vi "get_data_path.vi"(10 "Dataset directory":path=path "C:/Users/Naomi Tan/Documents/Gillette/ML/STIR_ML_dev/LabView/original_images/IMG_6155.JPG", 11 "Image path":path) -> (2 "Exists":bool, 3 "Dataset path":path)   [LabVIEW 2024]
panel:
  out "Exists 2":bool
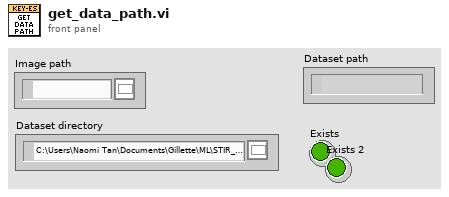
[diagram p1: front panel]
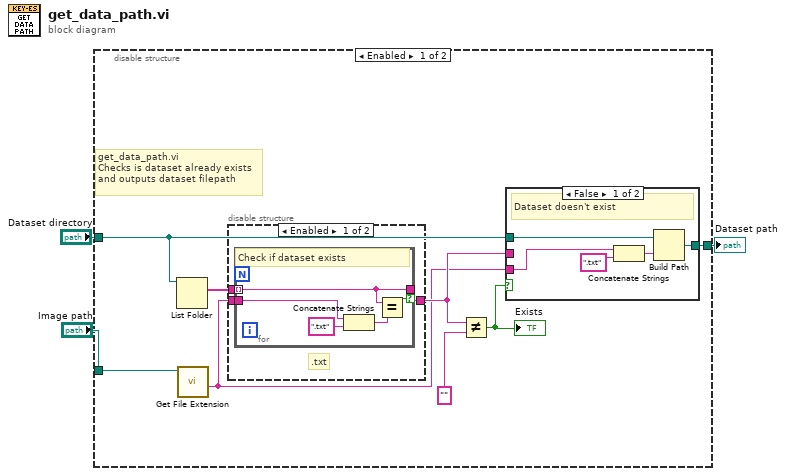
[diagram p0: block diagram]
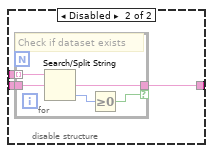
[diagram p2: hidden frame]
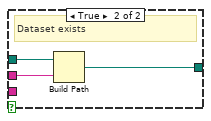
[diagram p3: hidden frame]
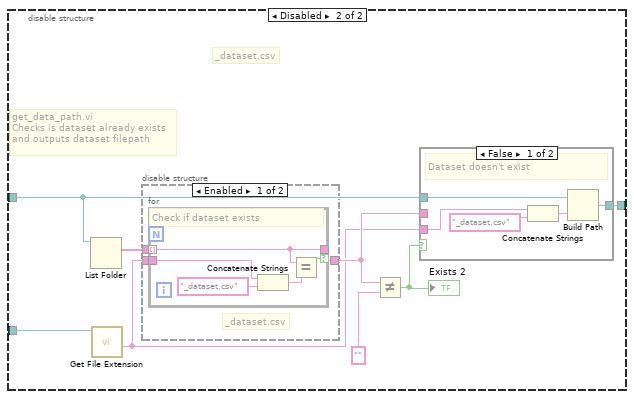
[diagram p4: hidden frame]
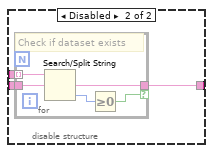
[diagram p5: hidden frame]
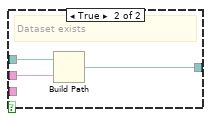
[diagram p6: hidden frame]
diagram:
  n1 = disable-structure shown="Enabled" {
    disable-tunnel: "Image path" -> [w11 w43]
    disable-tunnel: "Dataset directory" -> [w7 w39]
    disable-tunnel: [w4 w36] -> w1
    frame Enabled {
      # "get_data_path.vi\nChecks is dataset already exists\nand outputs dataset filepath"
      n2 = List Folder(path=w7) -> (filenames=w10:string[])  [unwired: 3 in, 3 out]
      n3 = call <vilib>:"Get File Extension.vi"("file"=w11) -> ("filename without extension"=w5:string)  [unwired: 6 in, 4 out]
      n4 = disable-structure shown="Enabled" {
        disable-tunnel: w10 -> [w14 w22]
        disable-tunnel: [w12 w21] -> w6
        disable-tunnel: w5 -> [w13 w20]
        frame Enabled {
          # ".txt"
          n5 = for {
            tunnel: w14 -> [w16] mode=indexing
            tunnel: w13 -> [w18]
            tunnel: [w16] -> w12 if=w15
            # "Check if dataset exists"
            n6 = Concatenate Strings(w18, ".txt" ("string")) -> (w17:string)
            n7 = Equal?(x=w16, y=w17) -> (x = y?=w15:bool)
          }
        }
        frame Disabled {
          n8 = for {
            tunnel: w22 -> [w26] mode=indexing
            tunnel: w20 -> [w27]
            tunnel: [w25] -> w21 if=w23
            # "Check if dataset exists"
            n9 = Search/Split String(string=w26, search string/char (-)=w27) -> (match + rest of string=w25:string, offset of match=w24:i32)  [unwired: 1 in, 1 out]
            n10 = Greater Or Equal To 0?(x=w24) -> (x >= 0?=w23:bool)
          }
        }
      }
      n11 = Not Equal?(x=w6, y="" ("delimiter (\\t)")) -> (x != y?=w8:bool)
      "Exists" <- w8
      n12 = case shown="False" w8 {
        tunnel: w7 -> [w32 w35]
        tunnel: w6 -> [_ w34]
        tunnel: w5 -> [w30 _]
        tunnel: [w28 w33] -> w4
        frame False {
          # "Dataset doesn't exist"
          n13 = Concatenate Strings(w30, ".txt" ("string")) -> (w31:string)
          n14 = Build Path(base path=w32, name or relative path=w31) -> (appended path=w28:path)
        }
        frame True {
          # "Dataset exists"
          n15 = Build Path(base path=w35, name or relative path=w34) -> (appended path=w33:path)
        }
      }
    }
    frame Disabled {
      # "_dataset.csv"
      # "get_data_path.vi\nChecks is dataset already exists\nand outputs dataset filepath"
      n16 = List Folder(path=w39) -> (filenames=w42:string[])  [unwired: 3 in, 3 out]
      n17 = call <vilib>:"Get File Extension.vi"("file"=w43) -> ("filename without extension"=w37:string)  [unwired: 6 in, 4 out]
      n18 = disable-structure shown="Enabled" {
        disable-tunnel: w42 -> [w46 w54]
        disable-tunnel: [w44 w53] -> w38
        disable-tunnel: w37 -> [w45 w52]
        frame Enabled {
          # "_dataset.csv"
          n19 = for {
            tunnel: w46 -> [w48] mode=indexing
            tunnel: w45 -> [w50]
            tunnel: [w48] -> w44 if=w47
            # "Check if dataset exists"
            n20 = Concatenate Strings(w50, "_dataset.csv" ("string")) -> (w49:string)
            n21 = Equal?(x=w48, y=w49) -> (x = y?=w47:bool)
          }
        }
        frame Disabled {
          n22 = for {
            tunnel: w54 -> [w58] mode=indexing
            tunnel: w52 -> [w59]
            tunnel: [w57] -> w53 if=w55
            # "Check if dataset exists"
            n23 = Search/Split String(string=w58, search string/char (-)=w59) -> (match + rest of string=w57:string, offset of match=w56:i32)  [unwired: 1 in, 1 out]
            n24 = Greater Or Equal To 0?(x=w56) -> (x >= 0?=w55:bool)
          }
        }
      }
      n25 = Not Equal?(x=w38, y="" ("delimiter (\\t)")) -> (x != y?=w40:bool)
      "Exists 2" <- w40
      n26 = case shown="False" w40 {
        tunnel: w39 -> [w64 w67]
        tunnel: w38 -> [_ w66]
        tunnel: w37 -> [w62 _]
        tunnel: [w60 w65] -> w36
        frame False {
          # "Dataset doesn't exist"
          n27 = Concatenate Strings(w62, "_dataset.csv" ("string")) -> (w63:string)
          n28 = Build Path(base path=w64, name or relative path=w63) -> (appended path=w60:path)
        }
        frame True {
          # "Dataset exists"
          n29 = Build Path(base path=w67, name or relative path=w66) -> (appended path=w65:path)
        }
      }
    }
  }
  "Dataset path" <- w1
